vi "DPT TC Panel Initial.vi"(10 "cDAQ index array":i32[][](array[numeric]), 11 "Array":string[][](array[string])) -> (0 "TC Panel 4":T1[][](array[typedef]), 1 "TC Panel 3":T1[][](array[typedef]), 2 "TC Panel 2":T1[][](array[typedef]), 3 "TC Panel 1":T1[][](array[typedef]))   [LabVIEW 2016]
doc: "Initialize TC Panel clusters"
uses:
  Type Definitions/DPT Channel Label.ctl
  Utility/Custom Pallet Controls/Custom Pallet String.ctl
panel:
  in  "Initialize":bool
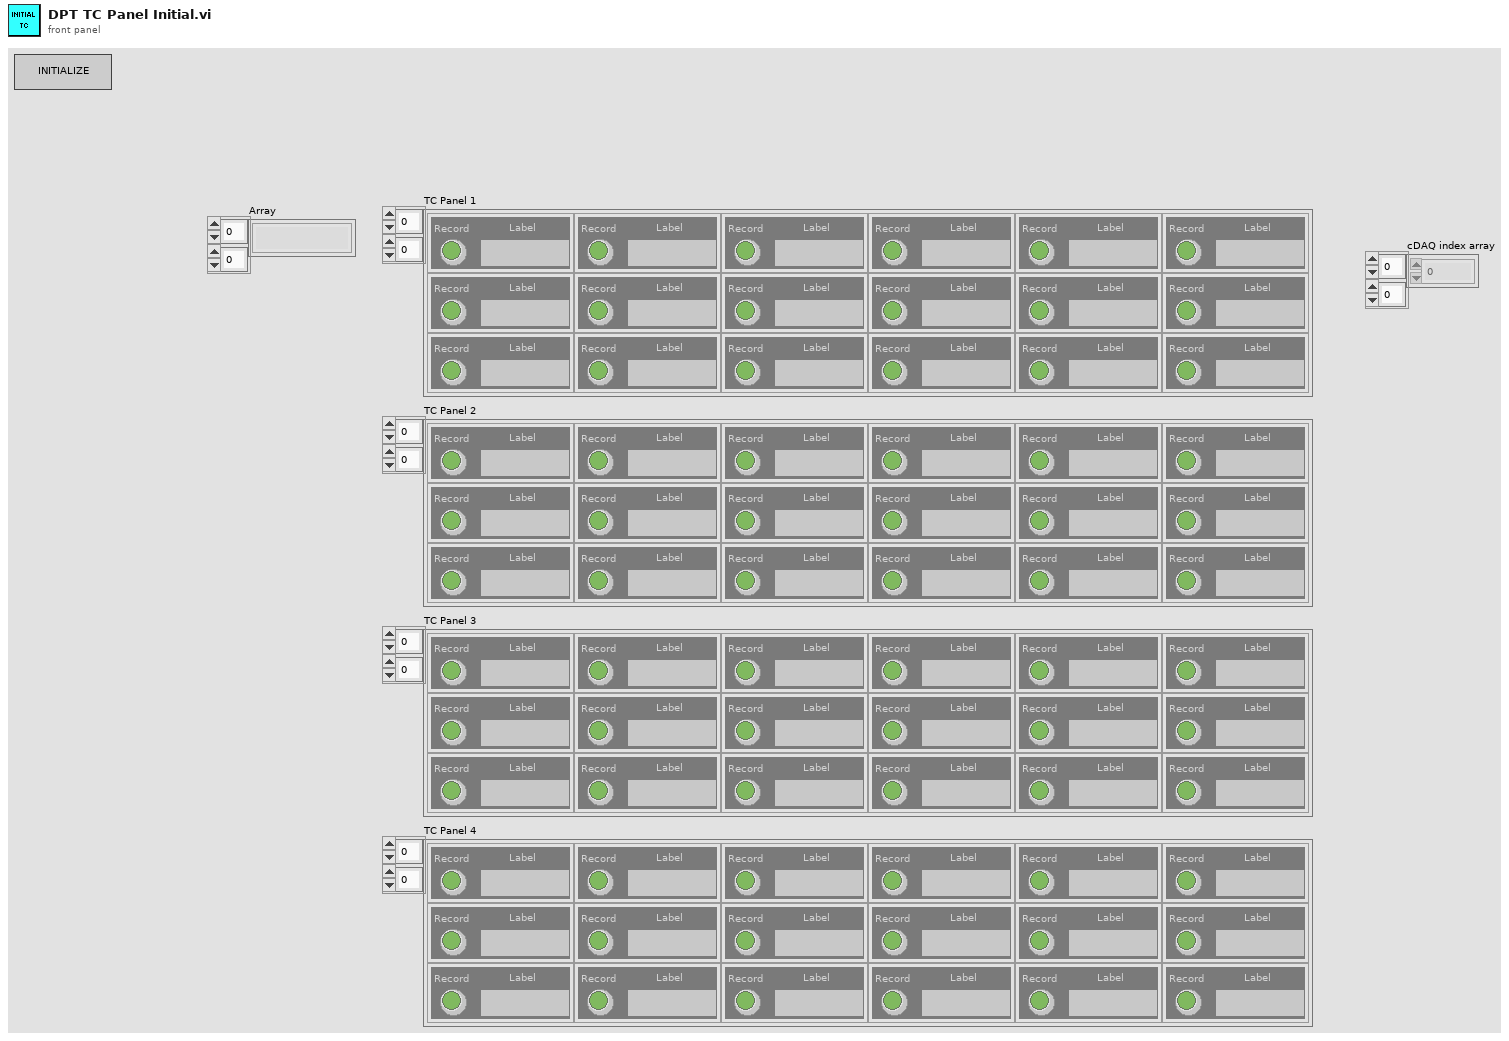
[diagram p1: front panel]
types:
  T1 = typedef "DPT Channel Label.ctl" = cluster{"Label":T2, "Record":bool, "Index":u32, "Channel":string}
  T2 = typedef "Custom Pallet String.ctl" = string
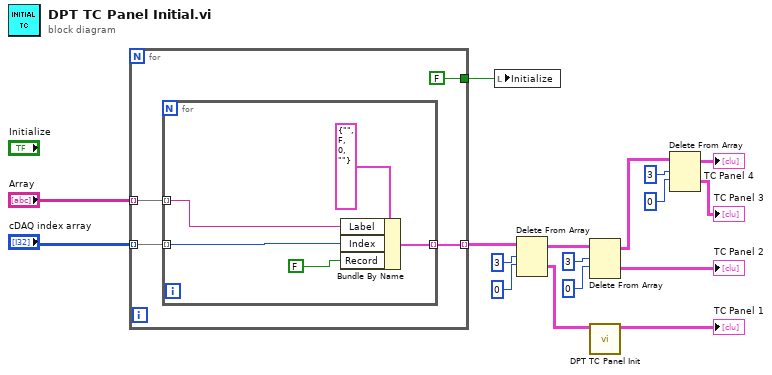
[diagram p0: block diagram]
diagram:
  n1 = for {
    tunnel: [w21] -> w17 mode=indexing
    tunnel: "Array" -> [w20] mode=indexing
    tunnel: "cDAQ index array" -> [w19] mode=indexing
    tunnel: [FALSE ("Read None")] -> w10
    n2 = for {
      tunnel: [w26] -> w21 mode=indexing
      tunnel: w20 -> [w25] mode=indexing
      tunnel: w19 -> [w24] mode=indexing
      n3 = Bundle By Name(cluster=T1 {"Label"="", "Record"=FALSE, "Index"=0, "Channel"=""} ("Sensor 2"), "Label"=w25, "Index"=w24, "Record"=FALSE ("Rec")) -> (w26:T1)
    }
  }
  n4 = local write "Initialize"(w10) -> ()
  n5 = Delete From Array(array=w17, length=3, index (row)=0) -> (deleted portion=w2:T1[][], array with subset deleted=w12:T1[][])  [unwired: 1 in]
  n6 = Delete From Array(array=w12, length=3, index (row)=0) -> (deleted portion=→"TC Panel 2":T1[][], array with subset deleted=w7:T1[][])  [unwired: 1 in]
  n7 = call "DPT TC Panel Init.vi"("TC Panel"=w2) -> ("TC Panel 1"=→"TC Panel 1":T1[][])  [unwired: 10 in]
  n8 = Delete From Array(array=w7, length=3, index (row)=0) -> (deleted portion=→"TC Panel 3":T1[][], array with subset deleted=→"TC Panel 4":T1[][])  [unwired: 1 in]
